vi "lvcsm String to Path.vi"(11 "Common Path":string) -> (3 "Path":path)   [LabVIEW 2017, in "lvcsm File Support.lvlib"]
uses:
  lvcsm File Support.lvlib
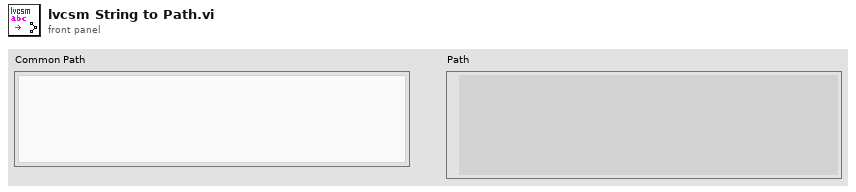
[diagram p1: front panel]
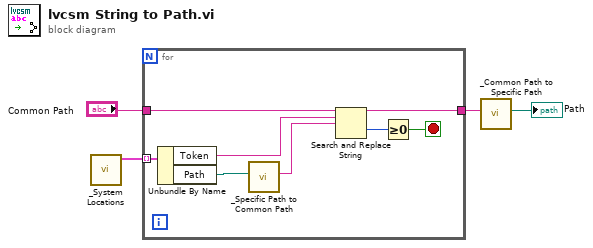
[diagram p0: block diagram]
diagram:
  n1 = call "_System Locations.vi"() -> ("SystemLocations"=w4:cluster{"Token":string, "Path":path}[])  [unwired: 11 in]
  n2 = for {
    tunnel: "Common Path" -> [w12]
    tunnel: [w11] -> w2
    tunnel: w4 -> [w8] mode=indexing
    stop <- w9 stop-if-true
    n3 = Unbundle By Name(w8) -> ("Token"=w6:string, "Path"=w7:path)
    n4 = call "_Specific Path to Common Path.vi"("Specific Path"=w7) -> ("Common Path"=w5:string)  [unwired: 10 in]
    n5 = Search and Replace String(input string=w12, search string=w6, replace string=w5) -> (result string=w11:string, offset past replacement=w10:i32)  [unwired: 5 in, 2 out]
    n6 = Greater Or Equal To 0?(x=w10) -> (x >= 0?=w9:bool)
  }
  n7 = call "_Common Path to Specific Path.vi"("Common Path"=w2) -> ("Specific Path"=→"Path":path)  [unwired: 10 in]
